vi "pylon_config.vi"(0 "?":T1={"X start"=0, "X end"=1023, "X Binning/Grouping"=1, "Y start"=0, "Y end"=1, "Y Binning/Grouping"=1}, 1 "Timing Mode":u16(ring) items=["Free Run", "Triger First", "Ext Sync", "Bulb Mode", "Variable Mode", "Flash Mode"], 2 "Logic Out":u16(ring) items=["Not Scan", "Shutter", "Not Rady", "Logic 0", "Clearing", "Not Ft Image Shift", "Reserved", "Logic1", "Expos Prog", "Expos", "Image Shift", "Readout", "Acquiring", "Wait For Trig"], 3 "Trigger Edge":u16(ring) items=["Positive", "Negative"], 4 "Use Custom Chip":bool, 5 "PyLonN Error In":errorcluster, 6 "Temperature":dbl=-100.0 caption="SET Temperature" format="%.2f", 8 "ADC Gain":u16(ring) items=["ADC Low", "ADC High"], 9 "Vertical Timing":dbl=3.2, 10 "ADC Speed":u16(ring)=2 items=["ADC Slowest"=0, "ADC Fastest"=1, "Default"=2, "50 kHz"=50, "100 kHz"=100, "200 kHz"=200, "500 kHz"=500, "1 MHz"=1000], 11 "Skip Serial  Reg Clean":dbl=1.0 format="%.2f", 12 "Readout Port":i32=4 min=-1 step=1, 16 "Shutter State":u16(ring)=2 items=["Always Close", "Open Each Exposure", "Open Until Finish", "Open waiting for triger"]) -> (13 "Vertical Timing":dbl, 14 "CameraHandle":u32, 18 "Readout Time":dbl caption="Readout time (ms)" format="%.2f", 19 "error out":errorcluster)   [LabVIEW 2014]
uses:
  Labview VIs/PIXIS_TEST/SITK_Labview/Examples70_2_2_0_1/RS Pixis/MaxY.vi
  Labview VIs/PIXIS_TEST/SITK_Labview/Examples70_2_2_0_1/RS Pixis/MaxX.vi
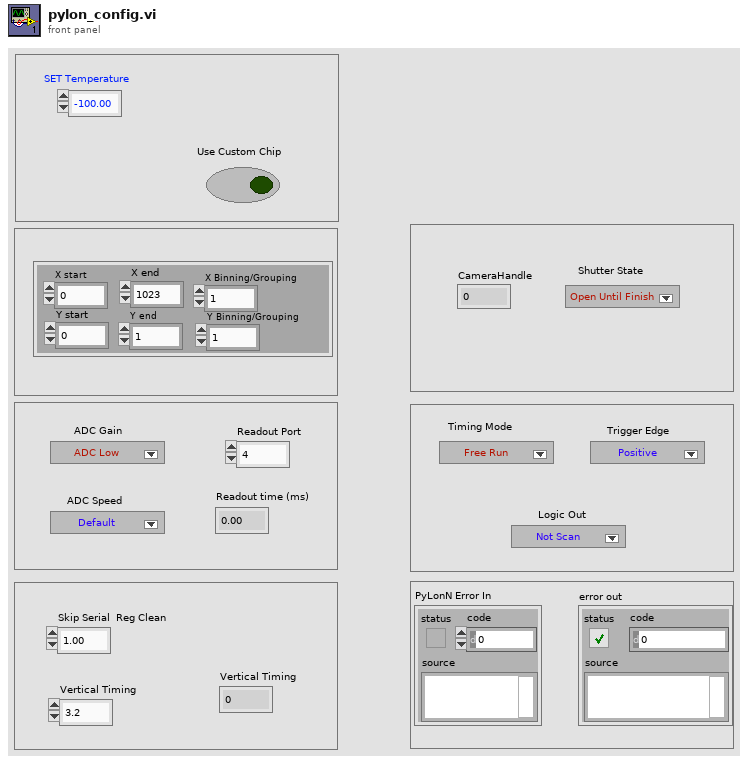
[diagram p1: front panel]
types:
  T1 = cluster{"X start":u32, "X end":u32, "X Binning/Grouping":u32, "Y start":u32, "Y end":u32, "Y Binning/Grouping":u32}
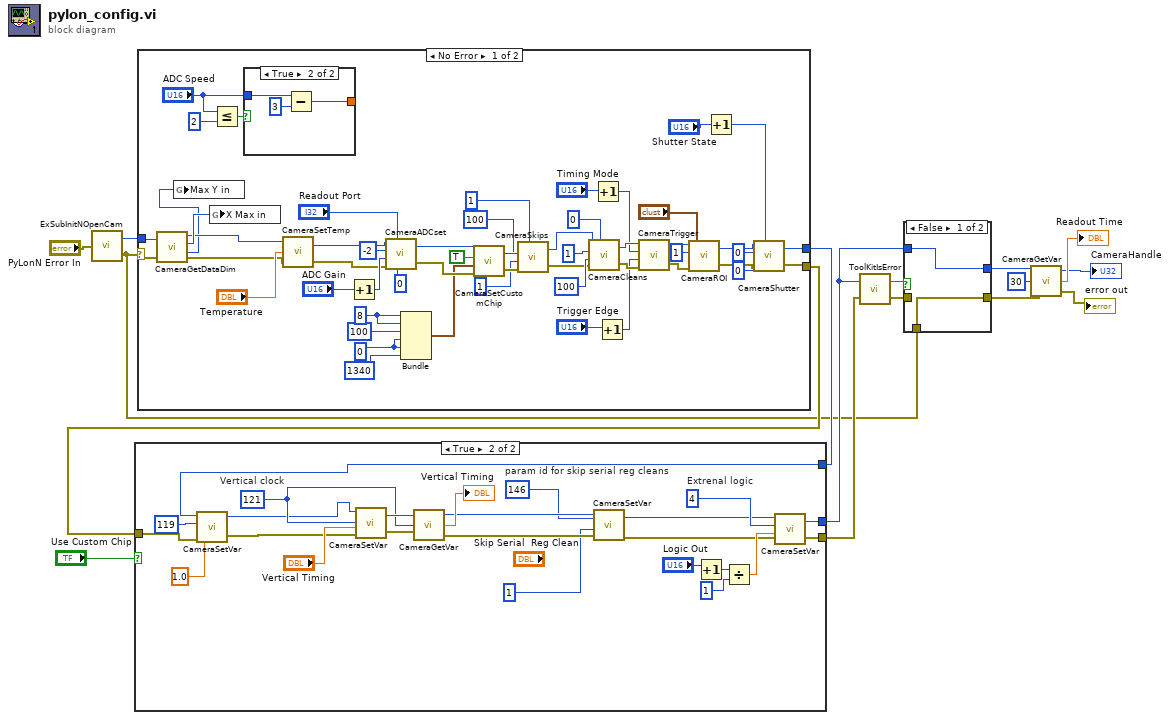
[diagram p0: block diagram]
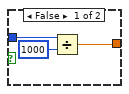
[diagram p4: hidden frame]
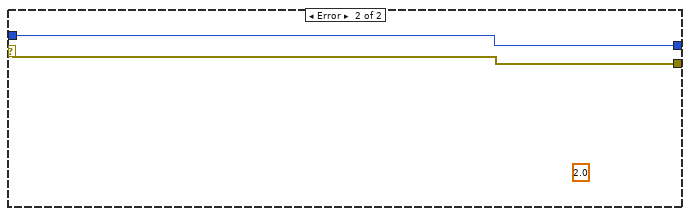
[diagram p5: hidden frame]
diagram:
  n1 = call "ExSubInitNOpenCam.vi"("error in (no error)"="PyLonN Error In") -> ("Camera Handle"=w15:u32, "error out"=w1:errorcluster)
  n2 = case shown="No Error" w1 {
    selector: w1 -> [w46 w76]
    tunnel: w15 -> [w28 w75]
    tunnel: [w18 w75] -> w14
    tunnel: [w20 w76] -> w9
    frame No Error {
      w43 = 0
      w45 = 8
      n3 = call <userlib>:"CameraGetDataDim.vi"("Camera Handle"=w28) -> ("Camera Handle"=w27:u32, "Xdim"=w29:u32, "Ydim"=w26:u32)  [unwired: 1 in, 1 out]
      n4 = global write "MaxY.vi" "Max Y in"(w26) -> ()
      n5 = global write "MaxX.vi" "X Max in"(w29) -> ()
      n6 = Less Or Equal?(x="ADC Speed", y=u16 2) -> (x <= y?=w51:bool)
      n7 = case shown="True" w51 {
        tunnel: "ADC Speed" -> [w71 w74]
        tunnel: [w69 w72] -> _
        frame False {
          n8 = Divide(x=w71, y=u16 1000) -> (x/y=w69:dbl)
        }
        frame True {
          n9 = Subtract(x=w74, y=u16 3) -> (x-y=w72:u16)
        }
      }
      n10 = call <userlib>:"CameraSetTemp.vi"("error in (no error)"=w46, "Temperature"="Temperature", "Camera Handle"=w27) -> ("error out"=w47:errorcluster, "Camera Handle"=w48:u32)
      n11 = Increment(x="ADC Gain") -> (x+1=w67:u16)
      n12 = call <userlib>:"CameraADCset.vi"("ADC offset"=0, "Read Out port"="Readout Port", "error in (no error)"=w47, "ADC Gain"=w67, "ADC Speed"=-2, "Camera Handle"=w48) -> ("error out"=w41:errorcluster, "Camera Handle"=w38:u32)
      n13 = Bundle(w45, w45, 100, w43, w43, 1340) -> (w40:cluster{i32, i32, i32, i32, i32, i32})  [unwired: 1 in]
      n14 = call <userlib>:"CameraSetCustomChip.vi"("error in (no error)"=w41, "Custom Chip Settings"=w40, "Enable/Disable Custom Chip"=TRUE, "Camera Handle"=w38) -> ("error out"=w35:errorcluster, "Camera Handle"=w37:u32)
      n15 = call <userlib>:"CameraSkips.vi"("Camera Handle"=w37, "Minimum Block Size"=u32 100, "Number of Minimum blocks"=u32 1, "error in"=w35, "Type of Skips"=u32 1) -> ("Camera Handle"=w36:u32, "error out"=w34:errorcluster)
      n16 = call <userlib>:"CameraCleans.vi"("Camera Handle"=w36, "Number of Clears"=u32 1, "Number of Strips Per Clear"=u32 100, "error in"=w34, "Continuous Clears"=u32 0) -> ("Camera Handle"=w65:u32, "error out"=w60:errorcluster)
      n17 = Increment(x="Timing Mode") -> (x+1=w54:u16)
      n18 = Increment(x="Trigger Edge") -> (x+1=w52:u16)
      n19 = call <userlib>:"CameraTrigger.vi"("error in"=w60, "Trigger Edge"=w52, "Timing Mode"=w54, "Camera Handle"=w65) -> ("error out"=w59:errorcluster, "Camera Handle"=w64:u32)
      n20 = call <userlib>:"CameraROI.vi"("error in"=w59, "ROI Params"="?", "ROI Index"=u32 1, "Camera Handle"=w64) -> ("error out"=w21:errorcluster, "Camera Handle"=w19:u32)
      n21 = Increment(x="Shutter State") -> (x+1=w17:u16)
      n22 = call <userlib>:"CameraShutter.vi"("Camera Handle"=w19, "Shutter Comp Time: Pre Open"=u32 0, "Shutter Comp Time: Post Open"=u32 0, "error in"=w21, "Shutter State"=w17) -> ("Camera Handle"=w18:u32, "error out"=w20:errorcluster)
    }
    frame Error {
      (unwired) 2.0 ("Value")
    }
  }
  n23 = case shown="True" "Use Custom Chip" {
    tunnel: w14 -> [w77 w82]
    tunnel: w9 -> [w78 w84]
    tunnel: [w77 w88] -> w10
    tunnel: [w78 w86] -> w11
    frame False {
    }
    frame True {
      w90 = 4  # Extrenal logic
      w96 = 146  # param id for skip serial reg cleans
      w101 = u32 121  # Vertical clock
      n24 = call <userlib>:"CameraSetVar.vi"("error in"=w84, "Value"=1.0, "Parameter ID"=u32 119, "Camera Handle"=w82) -> ("error out"=w83:errorcluster, "CameraHandle"=w81:u32)
      n25 = call <userlib>:"CameraSetVar.vi"("error in"=w83, "Value"="Vertical Timing", "Parameter ID"=w101, "Camera Handle"=w81) -> ("error out"=w100:errorcluster, "CameraHandle"=w102:u32)
      n26 = call <userlib>:"CameraGetVar.vi"("error in"=w100, "Parameter ID"=w101, "Camera Handle"=w102) -> ("error out"=w97:errorcluster, "Value"=→"Vertical Timing":dbl, "Camera Handle"=w98:u32)
      n27 = call <userlib>:"CameraSetVar.vi"("error in"=w97, "Value"=1, "Parameter ID"=w96, "Camera Handle"=w98) -> ("error out"=w87:errorcluster, "CameraHandle"=w89:u32)
      n28 = Increment(x="Logic Out") -> (x+1=w93:u16)
      n29 = Divide(x=w93, y=u16 1) -> (x/y=w91:dbl)
      n30 = call <userlib>:"CameraSetVar.vi"("error in"=w87, "Value"=w91, "Parameter ID"=w90, "Camera Handle"=w89) -> ("error out"=w86:errorcluster, "CameraHandle"=w88:u32)
    }
  }
  n31 = call <userlib>:"ToolKitIsError.vi"("error in"=w11, "Reserved"=w10) -> ("error out"=w12:errorcluster, "Error Flag"=w13:bool)
  n32 = case shown="False" w13 {
    tunnel: [w103 w106] -> w4
    tunnel: [w104 w105] -> w5
    tunnel: w12 -> [_ w106]
    tunnel: w10 -> [w104 w105]
    tunnel: w1 -> [w103 _]
    frame False {
    }
    frame True {
    }
  }
  n33 = call <userlib>:"CameraGetVar.vi"("error in"=w4, "Parameter ID"=u32 30, "Camera Handle"=w5) -> ("error out"=→"error out":errorcluster, "Value"=→"Readout Time":dbl, "Camera Handle"=→"CameraHandle":u32)
